vi "Convert data into CAN Frame type.vi"(8 "error in":errorcluster, 10 "Frame":string[](array[string])) -> (0 "error out":errorcluster, 2 "ID":u32, 3 "CAN frame":T1 {"payload" format="%x"; "timestamp" format="%<%.7X\n%x>T"; "type" items=["CAN Data"=0, "CAN Remote"=1, "CAN Bus Error"=2, "CAN 2.0 Data"=8, "CAN FD Data"=16, "CAN FD+BRS Data"=24, "J1939 Data"=192, "Delay"=224, "Log Trigger"=225, "Start Trigger"=226]; "identifier" format="%x"})   [LabVIEW 2025, in "CAN-LIN Raw Bus Capture UI.lvlib"]
doc: "This VI converts the DATA to CAN frame data type."
uses:
  CAN-LIN Raw Bus Capture UI.lvlib
  <vilib>/xnet/xnet.llb/XNET Frame CAN.ctl
  <vilib>/xnet/xnet.llb/XNET Frame Type CAN.ctl
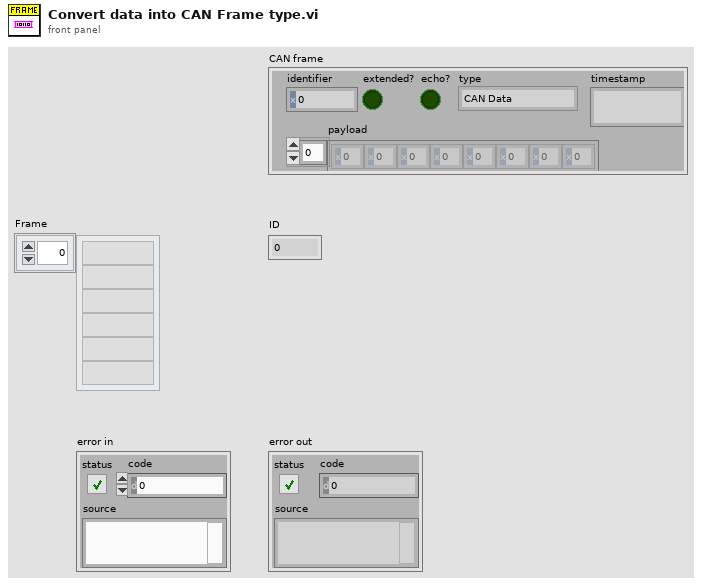
[diagram p1: front panel]
types:
  T1 = typedef "XNET Frame CAN.ctl" = cluster{"timestamp":timestamp, "payload":u8[], "identifier":u32, "type":T2, "extended?":bool, "echo?":bool}
  T2 = typedef "XNET Frame Type CAN.ctl" = u8
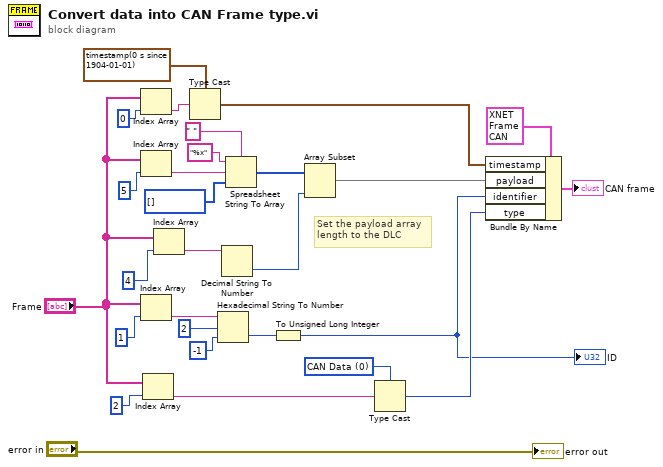
[diagram p0: block diagram]
diagram:
  w11 = T2 0 items=["CAN Data"=0, "CAN Remote"=1, "CAN Bus Error"=2, "CAN 2.0 Data"=8, "CAN FD Data"=16, "CAN FD+BRS Data"=24, "J1939 Data"=192, "Delay"=224, "Log Trigger"=225, "Start Trigger"=226] ("type")
  # "Set the payload array \nlength to the DLC"
  n1 = Index Array(array="Frame", index=0) -> (element=w18:string)
  n2 = Index Array(array="Frame", index=5) -> (element=w15:string)
  n3 = Index Array(array="Frame", index=1) -> (element=w23:string)
  n4 = Index Array(array="Frame", index=2) -> (element=w10:string)
  n5 = Index Array(array="Frame", index=4) -> (element=w5:string)
  n6 = Type Cast(type=timestamp(0 s since 1904-01-01) ("timestamp"), x=w18) -> (*(type *) &x=w27:timestamp)
  n7 = Hexadecimal String To Number(string=w23, offset=2, default (0uL)=-1 ("default (0 U32)")) -> (number=w20:i32)  [unwired: 1 out]
  n8 = Decimal String To Number(string=w5) -> (number=w3:i32)  [unwired: 2 in, 1 out]
  n9 = Spreadsheet String To Array(delimiter (Tab)=" ", format string="%x", spreadsheet string=w15, array type (2D Dbl)=u8[] [] ("payload")) -> (array=w4:u8[])
  n10 = To Unsigned Long Integer(number=w20) -> (unsigned 32bit integer=w8:u32)
  "ID" <- w8
  n11 = Array Subset(array=w4, length=w3) -> (w2:u8[])  [unwired: 1 in]
  n12 = Type Cast(type=w11, x=w10) -> (*(type *) &x=w9:T2)
  n13 = Bundle By Name(cluster=T1 {"timestamp"=timestamp(0 s since 1904-01-01), "payload"=[50, 32, 3, 0, 0], "identifier"=291, "type"=0, "extended?"=FALSE, "echo?"=FALSE} ("CAN frame"), "timestamp"=w27, "payload"=w2, "identifier"=w8, "type"=w9) -> (→"CAN frame":T1)
  "error out" <- "error in"
